vi "ABS.vi"() -> (2 "绝对模式":string)   [LabVIEW 2017]
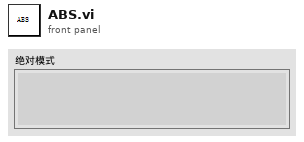
[diagram p1: front panel]
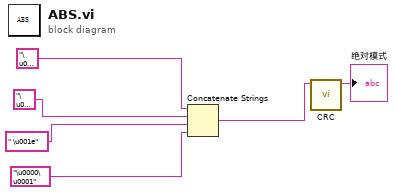
[diagram p0: block diagram]
diagram:
  n1 = Concatenate Strings("\u0001", "\u0006", " \u001e", "\u0000\u0001") -> (w5:string)
  n2 = call "CRC.vi"("字符串"=w5) -> ("连接的字符串"=→"绝对模式":string)  [unwired: 9 in, 1 out]
